vi "Msg.vi"(7 "jettl in":refnum<class "jettl.lvclass">, 11 "Override Error Msg Strategy in":refnum<class "Override Error Msg Strategy.lvclass">) -> (5 "jettl out":refnum<class "jettl.lvclass">)   [LabVIEW 2021, in "jettl.lvlib" / "Override Error.lvlib" / "Override Error Msg Strategy.lvclass"]
uses:
  Override Error Msg Strategy.lvclass
  jettl/jettl.lvclass
  Override Error/Override Error.lvclass
  Override Error Msg Strategy.lvclass/Override Error Msg Strategy.ctl
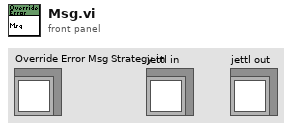
[diagram p1: front panel]
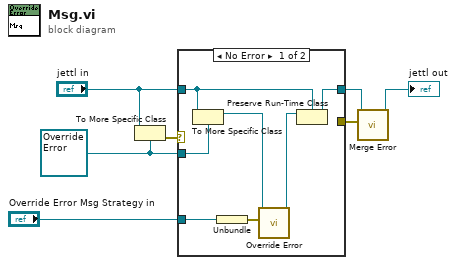
[diagram p0: block diagram]
diagram:
  w1 = refnum<class "Override Error.lvclass"> refnum ("jettl.lvlib:Override Error.lvlib:Override Error.lvclass")
  n1 = To More Specific Class(target class=w1, reference="jettl in") -> (error out=w7:errorcluster)  [unwired: 1 in, 1 out]
  n2 = case shown="No Error" w7 {
    selector: w7 -> [_ w15]
    tunnel: [w12 w16] -> w5
    tunnel: "jettl in" -> [w13 w16]
    tunnel: w1 -> [w14 _]
    tunnel: [_ w15] -> w6
    tunnel: "Override Error Msg Strategy in" -> [w9 _]
    frame No Error {
      n3 = To More Specific Class(target class=w14, reference=w13) -> (specific class reference=w10:refnum<class "Override Error.lvclass">)  [unwired: 1 in, 1 out]
      n4 = Unbundle(w9) -> (w8:errorcluster)
      n5 = call-dynamic "Override Error.vi"("Error"=w8, "Override Error in"=w10) -> ("Override Error out"=w11:refnum<class "Override Error.lvclass">)  [unwired: 9 in]
      n6 = Preserve Run-Time Class(object in=w11, 2:w13) -> (object out=w12:refnum<class "jettl.lvclass">)  [unwired: 1 in, 1 out]
    }
    frame Error {
    }
  }
  n7 = call-dynamic "Merge Error.vi"("Error"=w6, "Merge Error in"=w5) -> ("Merge Error out"=→"jettl out":refnum<class "jettl.lvclass">)  [unwired: 9 in]
